vi "Find Red Pitaya Lock-ins.vi"(6 "Timeout":i32=50, 7 "Acceptable logic tags":u16[](array[numeric])=[101, 102, 109, 110, 111, 112], 8 "Error In":errorcluster, 9 "End address":i32=110, 10 "Start address":i32=100, 11 "Subnet":string="192.168.1") -> (0 "Error Out":errorcluster, 1 "Addresses":string[](array[string]), 2 "Names":string[](array[string]), 3 "Instruments out":refnum<class "Instrument Actor.lvclass">[](array[class]))   [LabVIEW 2016]
uses:
  LabActor/Instrument Actor/Instrument Actor.lvclass
  LabActor/Recorders/Lock-in/Lock-in.lvclass
  C:/github/LabActor/Instrument Actor/Instrument Actor.lvclass
  Red Pitaya Lock-in Driver.lvclass
  C:/github/NHMFL_Core/Libraries/Instruments/Instrument Driver/Lock-in Driver/Lock-in Driver.lvclass
  Red Pitaya Lock-in Driver.lvclass/Red Pitaya Lock-in Driver.ctl
  Read RP Instrument.vi
  Write RP Instrument.vi
  RP Instrument/Write Server address.vi
  RP Instrument/Write Client type.vi
  LabActor/Recorders/Lock-in/Write Lock-in driver.vi
  RP Instrument/RP Instrument.lvclass
  Red Pitaya Digitizer/Red Pitaya Digitizer.lvclass
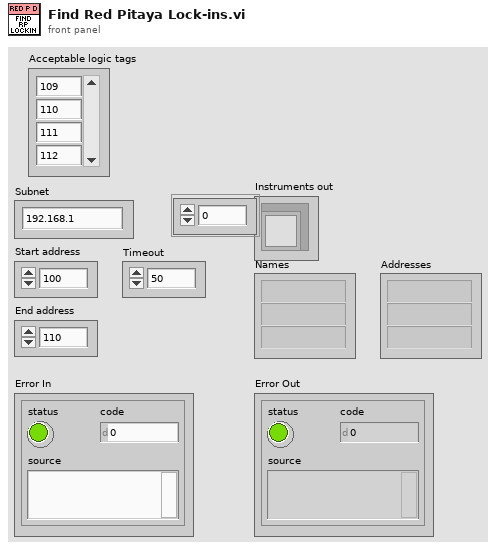
[diagram p1: front panel]
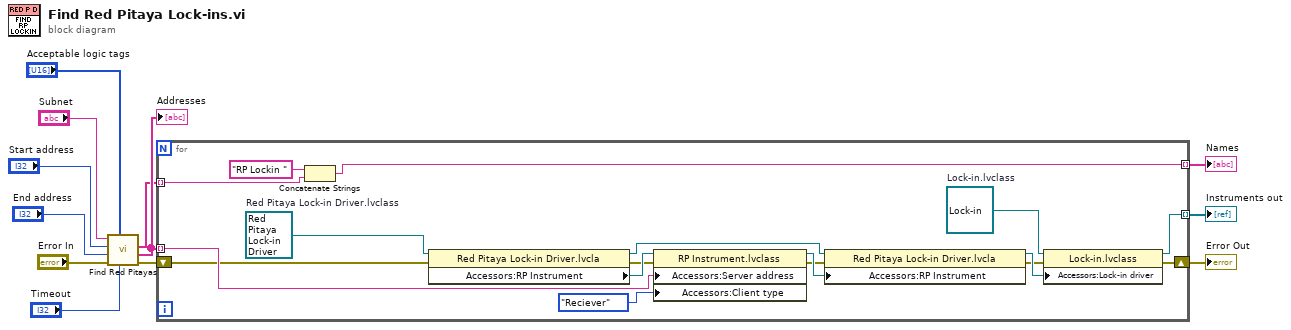
[diagram p0: block diagram]
diagram:
  n1 = call "Find Red Pitayas.vi"("Timeout"="Timeout", "Acceptable logic tags"="Acceptable logic tags", "Error In"="Error In", "End address"="End address", "Start address"="Start address", "Subnet"="Subnet") -> ("Error Out"=w6:errorcluster, "Addresses"=w7:string[], "Device names"=w2:string[])  [unwired: 2 in, 1 out]
  "Addresses" <- w7
  n2 = for {
    tunnel: w7 -> [w27] mode=indexing
    shift-right: [w18] -> w12
    shift-left: w6 -> [w25]
    tunnel: [w17] -> w3 mode=indexing
    tunnel: w2 -> [w15] mode=indexing
    tunnel: [w14] -> w1 mode=indexing
    w21 = refnum<class "Red Pitaya Lock-in Driver.lvclass"> refnum  # Red Pitaya Lock-in Driver.lvclass
    w22 = refnum<class "Lock-in.lvclass"> refnum  # Lock-in.lvclass
    n3 = Concatenate Strings("RP Lockin ", w15) -> (w14:string)
    n4 = property class="Red Pitaya Lock-in Driver.lvcla"(reference=w21, error in=w25) -> (reference out=w29:refnum<class "Red Pitaya Lock-in Driver.lvclass">, error out=w24:errorcluster, "Accessors:RP Instrument"=w28:refnum<class "RP Instrument.lvclass">)
    n5 = property class="RP Instrument.lvclass"(reference=w28, error in=w24, "Accessors:Server address"=w27, "Accessors:Client type"=enum16{"Control", "Reciever", "Transmitter"}."Reciever" ("Client type")) -> (reference out=w26:refnum<class "RP Instrument.lvclass">, error out=w23:errorcluster)
    n6 = property class="Red Pitaya Lock-in Driver.lvcla"(reference=w29, error in=w23, "Accessors:RP Instrument"=w26) -> (reference out=w20:refnum<class "Red Pitaya Lock-in Driver.lvclass">, error out=w19:errorcluster)
    n7 = property class="Lock-in.lvclass"(reference=w22, error in=w19, "Accessors:Lock-in driver"=w20) -> (reference out=w17:refnum<class "Lock-in.lvclass">, error out=w18:errorcluster)
  }
  "Instruments out" <- w3
  "Names" <- w1
  "Error Out" <- w12
